vi "ReshiftData.vi"(10 "TRIG_REC":u32, 11 "Data In":dbl[][](array[numeric])=array4x2560[10240 elements]) -> (3 "Data Out":dbl[][](array[numeric]))   [LabVIEW 2014]
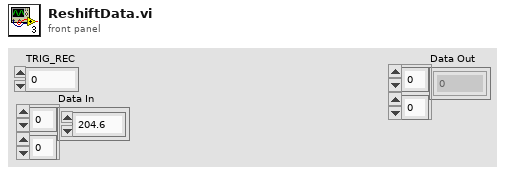
[diagram p1: front panel]
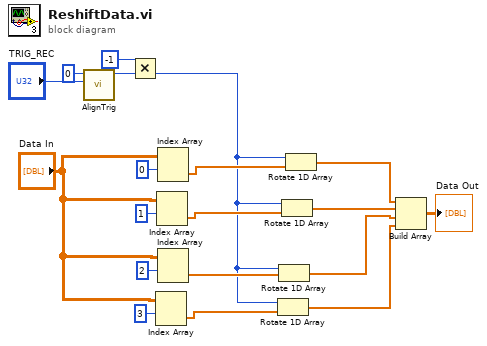
[diagram p0: block diagram]
diagram:
  n1 = call "AlignTrig.vi"("TRIG_REC"="TRIG_REC", "# Samples after Trig"=u16 0) -> ("Offset"=w8:i16)  [unwired: 9 in]
  n2 = Multiply(x=i16 -1, y=w8) -> (x*y=w2:i16)
  n3 = Index Array(array="Data In", index (row)=3) -> (element=w9:dbl[])  [unwired: 1 in]
  n4 = Index Array(array="Data In", index (row)=1) -> (element=w11:dbl[])  [unwired: 1 in]
  n5 = Index Array(array="Data In", index (row)=0) -> (element=w12:dbl[])  [unwired: 1 in]
  n6 = Index Array(array="Data In", index (row)=2) -> (element=w10:dbl[])  [unwired: 1 in]
  n7 = Rotate 1D Array(1:w9, 2:w2) -> (0:w4:dbl[])
  n8 = Rotate 1D Array(1:w10, 2:w2) -> (0:w5:dbl[])
  n9 = Rotate 1D Array(1:w11, 2:w2) -> (0:w6:dbl[])
  n10 = Rotate 1D Array(1:w12, 2:w2) -> (0:w7:dbl[])
  n11 = Build Array(w7, w6, w5, w4) -> (→"Data Out":dbl[][])
